vi "sandbox_simple.vi"() -> ()   [LabVIEW 2020]
panel:
  out "String":string
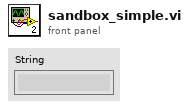
[diagram p1: front panel]
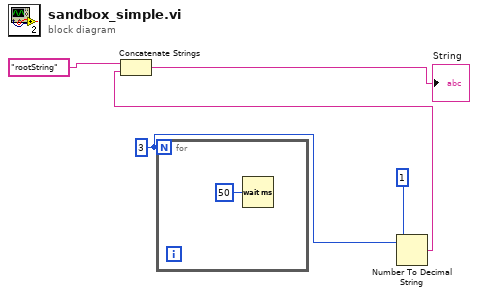
[diagram p0: block diagram]
diagram:
  w5 = 3
  n1 = for {
    N: w5 -> [_]
    n2 = Wait (ms)(milliseconds to wait=u32 50) -> ()  [unwired: 1 out]
  }
  n3 = Number To Decimal String(number=w5, width (-)=i16 1) -> (decimal integer string=w2:string)
  n4 = Concatenate Strings("rootString", w2) -> (→"String":string)
